vi "Build from database.vi"(8 "error in (no error)":errorcluster, 10 "Table Configuration":refnum<class "Table Configuration Interface.lvclass">, 11 "Table in":refnum<class "Table.lvclass">) -> (0 "error out":errorcluster, 3 "Table out":refnum<class "Table.lvclass">)   [LabVIEW 2020, in "Table.lvlib" / "Table.lvclass"]
uses:
  Table.lvclass
  Table Configuration Interface/Table Configuration Interface.lvclass
  Table.lvclass/Table.ctl
  Column Interface/Column Configuration Interface Class/Column Configuration.lvclass
  Database Interfaces/Database Interface Class/Database Interface.lvclass
  Column Factory/Column Factory.lvclass
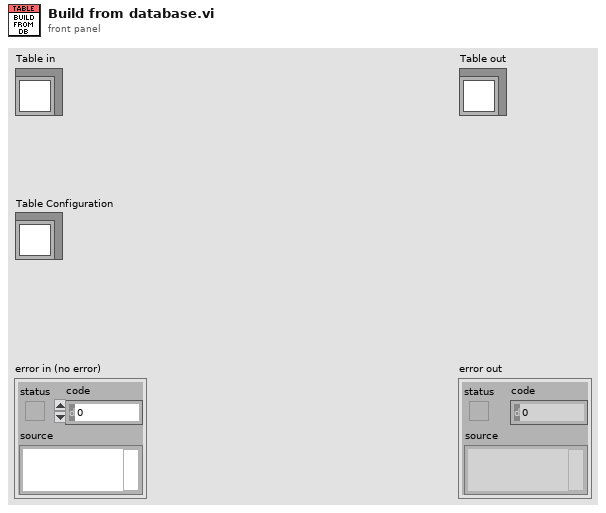
[diagram p1: front panel]
types:
  T1 = typedef "Database Interfaces.lvlib/Column Information.ctl" = cluster{"Name":string, "Type":T2, "Size (bytes)":i32}
  T2 = typedef "Database Interfaces.lvlib/Database data type.ctl" = enum16{"String", "Long (I32)", "Single (SGL)", "Double (DBL)", "Date/Time", "Binary"}
  T3 = map{string, refnum<class "Column Interface.lvclass">}
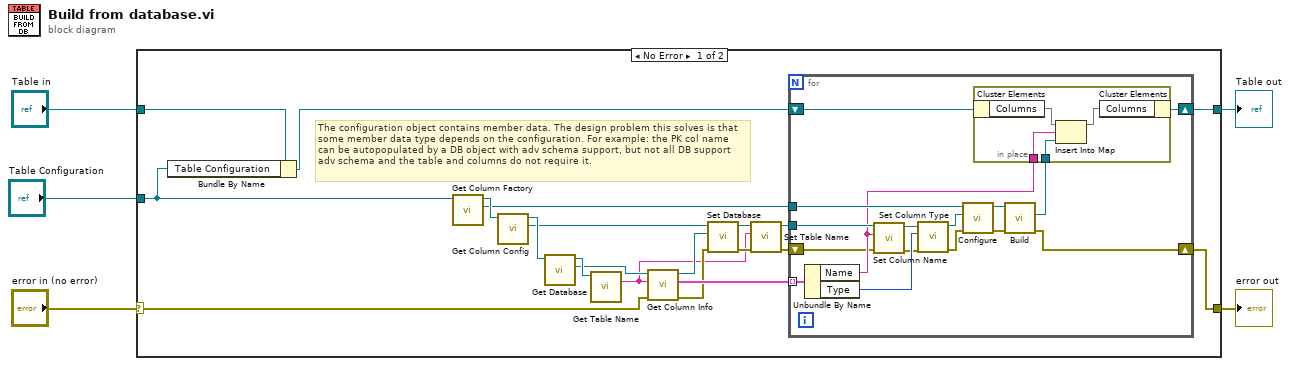
[diagram p0: block diagram]
diagram:
  n1 = case shown="No Error" "error in (no error)" {
    selector: "error in (no error)" -> [w19 w47]
    tunnel: [w16 w47] -> w4
    tunnel: [w17 w46] -> w2
    tunnel: "Table in" -> [w8 w46]
    tunnel: "Table Configuration" -> [w6 _]
    frame No Error {
      # "The configuration object contains member data. The design problem this solves is that some member data type depends on the configuration. For example: the PK col name can be autopopulated by a DB object with adv schema support, but not all DB support adv schema and the table and columns do not require it."
      n2 = Bundle By Name(cluster=w8, "Table Configuration"=w6) -> (w7:refnum<class "Table.lvclass">)
      n3 = call-dynamic "Get Column Factory.vi"("Table Configuration Interface in"=w6) -> ("Column Factory"=w12:refnum<class "Column Factory.lvclass">, "Table Configuration Interface out"=w15:refnum<class "Table Configuration Interface.lvclass">)  [unwired: 8 in, 1 out]
      n4 = call-dynamic "Get Column Config.vi"("Table Configuration Interface in"=w15) -> ("Column Configuration"=w11:refnum<class "Column Configuration.lvclass">, "Table Configuration Interface out"=w14:refnum<class "Table Configuration Interface.lvclass">)  [unwired: 8 in, 1 out]
      n5 = call-dynamic "Get Database.vi"("Table Configuration Interface in"=w14) -> ("Database"=w10:refnum<class "Database Interface.lvclass">, "Table Configuration Interface out"=w13:refnum<class "Table Configuration Interface.lvclass">)  [unwired: 8 in, 1 out]
      n6 = call-dynamic "Get Table Name.vi"("Table Configuration Interface in"=w13) -> ("Table Name"=w9:string)  [unwired: 8 in, 2 out]
      n7 = call-dynamic "Get Column Info.vi"("error in (no error)"=w19, "Table Name"=w9, "Database Interface in"=w10) -> ("error out"=w22:errorcluster, "Column Information Array"=w25:T1[], "Database Interface out"=w18:refnum<class "Database Interface.lvclass">)  [unwired: 6 in]
      n8 = call-dynamic "Set Database.vi"("error in (no error)"=w22, "Database"=w18, "Column Configuration in"=w11) -> ("error out"=w21:errorcluster, "Column Configuration out"=w24:refnum<class "Column Configuration.lvclass">)  [unwired: 7 in]
      n9 = call-dynamic "Set Table Name.vi"("error in (no error)"=w21, "Table Name"=w9, "Column Configuration in"=w24) -> ("error out"=w20:errorcluster, "Column Configuration out"=w23:refnum<class "Column Configuration.lvclass">)  [unwired: 7 in]
      n10 = for {
        tunnel: w25 -> [w41] mode=indexing
        tunnel: w23 -> [w39]
        tunnel: w12 -> [w36]
        shift-right: [w33] -> w17
        shift-left: w7 -> [w34]
        shift-right: [w26] -> w16
        shift-left: w20 -> [w30]
        n11 = Unbundle By Name(w41) -> ("Name"=w31:string, "Type"=w40:T2)
        n12 = call-dynamic "Set Column Name.vi"("error in (no error)"=w30, "Column Name"=w31, "Column Configuration in"=w39) -> ("error out"=w29:errorcluster, "Column Configuration out"=w38:refnum<class "Column Configuration.lvclass">)  [unwired: 7 in]
        n13 = call-dynamic "Set Column Type.vi"("error in (no error)"=w29, "Column Type"=w40, "Column Configuration in"=w38) -> ("error out"=w28:errorcluster, "Column Configuration out"=w37:refnum<class "Column Configuration.lvclass">)  [unwired: 7 in]
        n14 = call-dynamic "Configure.vi"("error in (no error)"=w28, "Configuration"=w37, "Column Factory in"=w36) -> ("error out"=w27:errorcluster, "Column Factory out"=w35:refnum<class "Column Factory.lvclass">)  [unwired: 7 in]
        n15 = call-dynamic "Build.vi"("error in (no error)"=w27, "Column Factory in"=w35) -> ("error out"=w26:errorcluster, "Column"=w32:refnum<class "Column Interface.lvclass">)  [unwired: 7 in, 1 out]
        n16 = in-place {
          in-place-border: w32 -> [w43]
          in-place-border: w31 -> [w42]
          n17 = in-place-cluster #1(w34) -> ("Columns"=w45:T3)
          n18 = Insert Into Map(map in=w45, key=w42, value=w43) -> (map out=w44:T3)  [unwired: 2 out]
          n19 = in-place-cluster #1("Columns"=w44) -> (w33:refnum<class "Table.lvclass">)
        }
      }
    }
    frame Error {
    }
  }
  "error out" <- w4
  "Table out" <- w2
